vi "Current-WL.vi"(2 "Boolean":bool, 3 "VISA resource name":refnum<visa-resource-name>="COM4") -> (0 "nm":dbl format="%.2f", 1 "cm-1":dbl format="%#_7g")   [LabVIEW 2018]
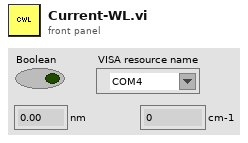
[diagram p1: front panel]
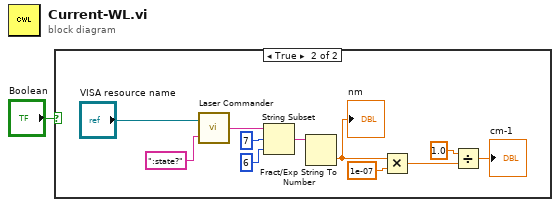
[diagram p0: block diagram]
diagram:
  n1 = case shown="True" "Boolean" {
    frame False {
    }
    frame True {
      n2 = call "Laser Commander.vi"("Laser Command"=":state?", "VISA resource name"="VISA resource name") -> ("Laser Response"=w4:string)
      n3 = String Subset(string=w4, offset (0)=7, length (rest)=6) -> (substring=w10:string)
      n4 = Fract/Exp String To Number(string=w10) -> (number=w5:dbl)  [unwired: 3 in, 1 out]
      "nm" <- w5
      n5 = Multiply(x=w5, y=1e-07) -> (x*y=w8:dbl)
      n6 = Divide(x=1.0, y=w8) -> (x/y=→"cm-1":dbl)
    }
  }
